vi "test-quintic-spline-04.vi"() -> ()   [LabVIEW 2019]
uses:
  <vilib>/Rock Robotics/WPI/ThirdParty/JAS_Junk/TrajLib/POSEwCURVATURE.ctl
  <vilib>/Rock Robotics/WPI/ThirdParty/JAS_Junk/TrajLib/POSE2D.ctl
  <vilib>/Rock Robotics/WPI/ThirdParty/JAS_Junk/TrajLib/TRANSLATION2D.ctl
  <vilib>/Rock Robotics/WPI/ThirdParty/JAS_Junk/TrajLib/ROTATION2D.ctl
  <vilib>/Rock Robotics/WPI/ThirdParty/JAS_Junk/TrajLib/Rotation_CreateAngle.vi
  <vilib>/Rock Robotics/WPI/ThirdParty/JAS_Junk/TrajLib/Translation_Create.vi
  <vilib>/Rock Robotics/WPI/ThirdParty/JAS_Junk/TrajLib/Util_CalcDist.vi
  <vilib>/Rock Robotics/WPI/ThirdParty/JAS_Junk/TrajLib/Trajectory_Library.lvlib
panel:
  out "XY Graph":cluster{dbl[], dbl[]}(graph)
  out "Numb\nWaypoints":i32
  out "All Interior \nwayPoints\nFound (True)":bool
  out "end rot = 0":dbl
  out "end y = 0":dbl
  out "end x = 0":dbl
  out "start rot = 0":dbl
  out "start y = 0":dbl
  out "start x = 0":dbl
  out "max dtheta < 0.0872":dbl
  out "max dy < 0.00127":dbl
  out "max dx  < 0.127":dbl
  out "Overall Error":errorcluster
  out "Elements":i32
  out "Create Spline Error":errorcluster
  out "SplinePoses\nWCurve":T1[](array[typedef]) {"POSE"."ROTATION"."SIN" format="%13.4f"; "POSE"."ROTATION"."COS" format="%13.4f"; "POSE"."ROTATION"."VALUE" format="%13.4f"; "POSE"."TRANSLATION"."Y" format="%14.3f"; "POSE"."TRANSLATION"."X" format="%14.3f"}
  out "Elapsed Time":dbl
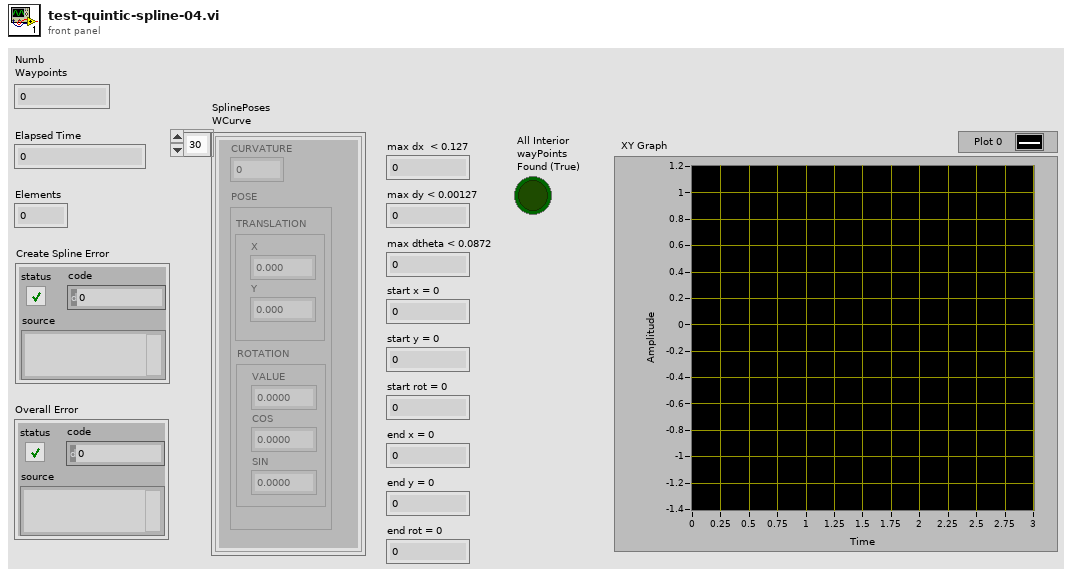
[diagram p1: front panel]
types:
  T1 = typedef "Trajectory_Library.lvlib/POSEwCURVATURE.ctl" = cluster{"CURVATURE":dbl, "POSE":T2}
  T2 = typedef "Trajectory_Library.lvlib/POSE2D.ctl" = cluster{"TRANSLATION":T3, "ROTATION":T4}
  T3 = typedef "Trajectory_Library.lvlib/TRANSLATION2D.ctl" = cluster{"X":dbl, "Y":dbl}
  T4 = typedef "Trajectory_Library.lvlib/ROTATION2D.ctl" = cluster{"VALUE":dbl, "COS":dbl, "SIN":dbl}
  T5 = typedef "Trajectory_Library.lvlib/SPLINE_CTRL_VECTOR.ctl" = cluster{"Xs":dbl[], "Ys":dbl[]}
  T6 = typedef "Trajectory_Library.lvlib/SPLINE.ctl" = cluster{"Degree":i32, "Coefficients":T7}
  T7 = typedef "NI_Matrix.lvlib/RealMatrix.ctl" = dbl[][]
  T8 = typedef "Trajectory_Library.lvlib/TWIST2D.ctl" = cluster{"dX":dbl, "dY":dbl, "dTHETA":dbl}
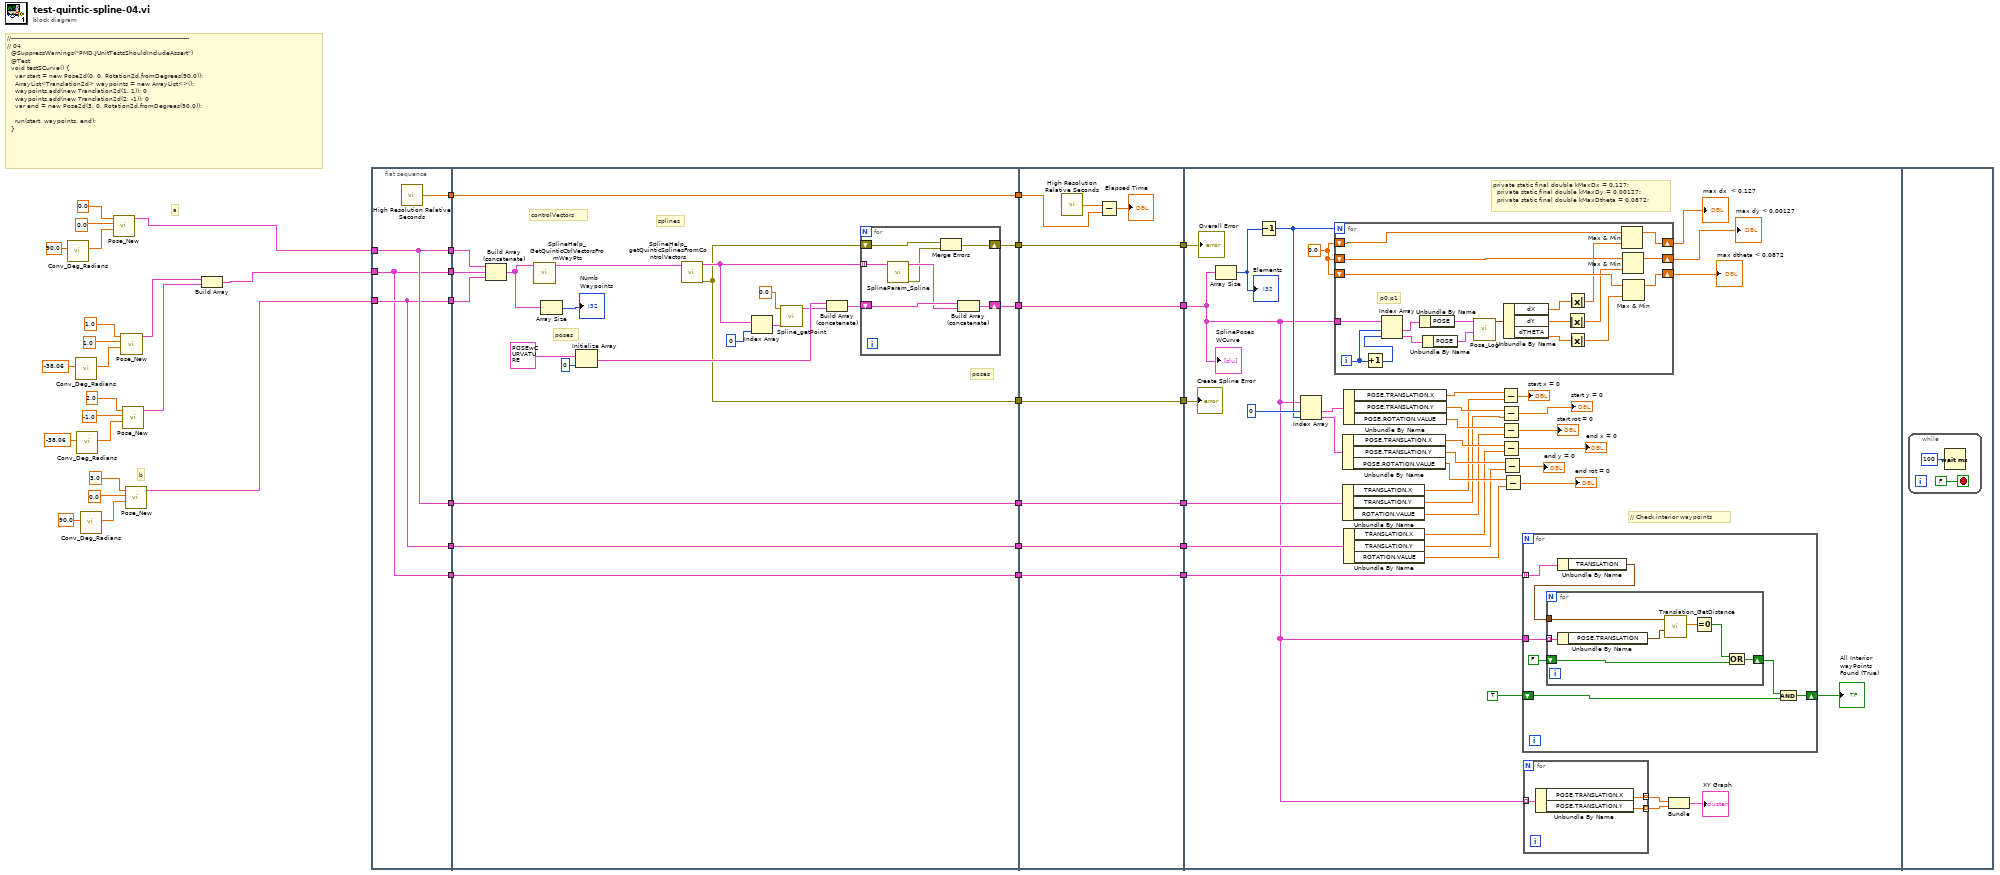
[diagram p0: block diagram]
diagram:
  # "b"
  # "a"
  # "//-----------------------------------------------------------------------------------------\n// 04\n  @SuppressWarnings(\"PMD.JUnitTestsShouldIncludeAssert\")\n  @Test\n  void testSCurve() {\n    var start = new Pose2d(0, 0, Rotation2d.fromDegrees(90.0));\n    ArrayList<Translation2d> waypoints = new ArrayList<>();\n    waypoints.add(new Translation2d(1, 1)); 0\n    waypoints.add(new Translation2d(2, -1)); 0\n    var end = new Pose2d(3, 0, Rotation2d.fromDegrees(90.0));\n\n    run(start, waypoints, end);\n  }"
  n1 = call <vilib>:"Conv_Deg_Radians.vi"("Degress"=90.0) -> ("Radians"=w15:dbl)  [unwired: 10 in]
  n2 = call <vilib>:"Conv_Deg_Radians.vi"("Degress"=-38.06) -> ("Radians"=w8:dbl)  [unwired: 10 in]
  n3 = call <vilib>:"Conv_Deg_Radians.vi"("Degress"=-38.06) -> ("Radians"=w4:dbl)  [unwired: 10 in]
  n4 = call <vilib>:"Conv_Deg_Radians.vi"("Degress"=90.0) -> ("Radians"=w18:dbl)  [unwired: 10 in]
  n5 = call <vilib>:"Pose_New.vi"("Heading"=w15, "Y"=0.0, "X"=0.0) -> ("out POSe"=w12:T2)  [unwired: 8 in]
  n6 = call <vilib>:"Pose_New.vi"("Heading"=w8, "Y"=1.0, "X"=1.0) -> ("out POSe"=w2:T2)  [unwired: 8 in]
  n7 = call <vilib>:"Pose_New.vi"("Heading"=w4, "Y"=-1.0, "X"=2.0) -> ("out POSe"=w1:T2)  [unwired: 8 in]
  n8 = call <vilib>:"Pose_New.vi"("Heading"=w18, "Y"=0.0, "X"=3.0) -> ("out POSe"=w40:T2)  [unwired: 8 in]
  n9 = Build Array(w2, w1) -> (w11:T2[])
  n10 = flat-sequence {
    tunnel: w12 -> [w44]
    tunnel: [w44] -> w41
    tunnel: w40 -> [w43]
    tunnel: [w43] -> w39
    tunnel: [w45] -> w38
    tunnel: [w44] -> w30
    tunnel: [w43] -> w27
    tunnel: [w42] -> w22
    tunnel: w11 -> [w42]
    tunnel: [w42] -> w21
    tunnel: w41 -> [w51]
    tunnel: w39 -> [w49]
    tunnel: [w67] -> w37
    tunnel: w38 -> [w67]
    tunnel: [w57] -> w36
    tunnel: [w56] -> w34
    tunnel: [w55] -> w32
    tunnel: w30 -> [w54]
    tunnel: [w54] -> w29
    tunnel: w27 -> [w53]
    tunnel: [w53] -> w26
    tunnel: [w52] -> w23
    tunnel: w22 -> [w52]
    tunnel: w21 -> [w48]
    tunnel: w37 -> [w83]
    tunnel: w36 -> [w82]
    tunnel: [w82] -> w35
    tunnel: w34 -> [w81]
    tunnel: [w81] -> w33
    tunnel: w32 -> [w80]
    tunnel: [w80] -> w31
    tunnel: w29 -> [w77]
    tunnel: [w77] -> w28
    tunnel: w26 -> [w76]
    tunnel: [w76] -> w25
    tunnel: [w75] -> w24
    tunnel: w23 -> [w75]
    tunnel: w35 -> [w85]
    tunnel: w33 -> [w121]
    tunnel: w31 -> [w120]
    tunnel: w28 -> [w114]
    tunnel: w25 -> [w113]
    tunnel: w24 -> [w90]
    frame #0 {
      n11 = call <vilib>:"High Resolution Relative Seconds.vi"() -> ("relative seconds"=w45:dbl)
    }
    frame #1 {
      # "poses"
      # "poses"
      # "splines"
      # "controlVectors"
      n12 = Build Array (concatenate)(w51, w48, w49) -> (w47:T2[])
      n13 = call <vilib>:"SplineHelp_GetQuinticCtrlVectorsFromWayPts.vi"("WayPoints"=w47) -> ("SplineControlVectors"=w50:T5[])  [unwired: 10 in]
      n14 = Array Size(array=w47) -> (size(s)=→"Numb\nWaypoints":i32)
      n15 = Initialize Array(T1 {"CURVATURE"=0.0, "POSE"={"TRANSLATION"={"X"=0.0, "Y"=0.0}, "ROTATION"={"VALUE"=0.0, "COS"=1.0, "SIN"=0.0}}} ("POSEwCURVATURE"), 0 ("dimension size")) -> (w61:T1[])
      n16 = call <vilib>:"SplineHelp_getQuinticSplinesFromControlVectors.vi"("ControlVectors"=w50) -> ("error out"=w56:errorcluster, "splines"=w58:T6[])  [unwired: 9 in]
      n17 = Index Array(array=w58, index=0) -> (element=w63:T6)
      n18 = call <vilib>:"Spline_getPoint.vi"("inputSPLINE"=w63, "Time"=0.0) -> ("POSEwCURVATURE"=w60:T1)  [unwired: 9 in]
      n19 = Build Array (concatenate)(w61, w60) -> (w59:T1[])
      n20 = for {
        shift-right: [w71] -> w57
        shift-left: w59 -> [w73]
        tunnel: w58 -> [w74] mode=indexing
        shift-right: [w69] -> w55
        shift-left: w56 -> [w70]
        n21 = call <vilib>:"SplineParam_Spline.vi"("inputSPLINE"=w74) -> ("error out"=w68:errorcluster, "outputPOSEwCURVATURE"=w72:T1[])  [unwired: 9 in]
        n22 = Merge Errors(w70, w68) -> (w69:errorcluster)
        n23 = Build Array (concatenate)(w73, w72) -> (w71:T1[])
      }
    }
    frame #2 {
      n24 = call <vilib>:"High Resolution Relative Seconds.vi"() -> ("relative seconds"=w78:dbl)
      n25 = Subtract(x=w78, y=w83) -> (x-y=→"Elapsed Time":dbl)
    }
    frame #3 {
      w118 = 0.0
      # "// Check interior waypoints"
      # "private static final double kMaxDx = 0.127;\n  private static final double kMaxDy = 0.00127;\n  private static final double kMaxDtheta = 0.0872;"
      n26 = Array Size(array=w85) -> (size(s)=w119:i32)
      "Elements" <- w119
      n27 = Decrement(x=w119) -> (x-1=w111:i32)
      n28 = Index Array(array=w85, index #1=0 ("index"), index #2=w111) -> (element #1=w110:T1, element #2=w109:T1)
      n29 = for {
        N: w111 -> [_]
        tunnel: w85 -> [w156]
        shift-right: [w147] -> w117
        shift-left: w118 -> [w144]
        shift-right: [w145] -> w115
        shift-left: w118 -> [w142]
        shift-right: [w146] -> w116
        shift-left: w118 -> [w143]
        i -> [w158]
        # "p0,p1"
        n30 = Increment(x=w158) -> (x+1=w157:i32)
        n31 = Index Array(array=w156, index #1=w158, index #2=w157) -> (element #1=w155:T1, element #2=w154:T1)
        n32 = Unbundle By Name(w155) -> ("POSE"=w153:T2)
        n33 = Unbundle By Name(w154) -> ("POSE"=w152:T2)
        n34 = call <vilib>:"Pose_Log.vi"("end POSE"=w152, "in POSE"=w153) -> ("out TWIST"=w151:T8)  [unwired: 9 in]
        n35 = Unbundle By Name(w151) -> ("dX"=w148:dbl, "dY"=w149:dbl, "dTHETA"=w150:dbl)
        n36 = Absolute Value(x=w149) -> (abs(x)=w140:dbl)
        n37 = Absolute Value(x=w148) -> (abs(x)=w141:dbl)
        n38 = Absolute Value(x=w150) -> (abs(x)=w139:dbl)
        n39 = Max & Min(x=w144, y=w141) -> (max(x,y)=w147:dbl)  [unwired: 1 out]
        n40 = Max & Min(x=w143, y=w140) -> (max(x,y)=w146:dbl)  [unwired: 1 out]
        n41 = Max & Min(x=w142, y=w139) -> (max(x,y)=w145:dbl)  [unwired: 1 out]
      }
      "max dx  < 0.127" <- w117
      "max dy < 0.00127" <- w116
      "max dtheta < 0.0872" <- w115
      n42 = Unbundle By Name(w109) -> ("POSE.TRANSLATION.X"=w105:dbl, "POSE.TRANSLATION.Y"=w104:dbl, "POSE.ROTATION.VALUE"=w103:dbl)
      n43 = Unbundle By Name(w114) -> ("TRANSLATION.X"=w102:dbl, "TRANSLATION.Y"=w101:dbl, "ROTATION.VALUE"=w100:dbl)
      n44 = Unbundle By Name(w110) -> ("POSE.TRANSLATION.X"=w108:dbl, "POSE.TRANSLATION.Y"=w107:dbl, "POSE.ROTATION.VALUE"=w106:dbl)
      n45 = Unbundle By Name(w113) -> ("TRANSLATION.X"=w99:dbl, "TRANSLATION.Y"=w98:dbl, "ROTATION.VALUE"=w97:dbl)
      n46 = Subtract(x=w108, y=w102) -> (x-y=→"start x = 0":dbl)
      n47 = Subtract(x=w107, y=w101) -> (x-y=→"start y = 0":dbl)
      n48 = Subtract(x=w106, y=w100) -> (x-y=→"start rot = 0":dbl)
      n49 = Subtract(x=w105, y=w99) -> (x-y=→"end x = 0":dbl)
      n50 = Subtract(x=w104, y=w98) -> (x-y=→"end y = 0":dbl)
      n51 = Subtract(x=w103, y=w97) -> (x-y=→"end rot = 0":dbl)
      n52 = for {
        tunnel: w90 -> [w126] mode=indexing
        tunnel: w85 -> [w131]
        shift-right: [w130] -> w88
        shift-left: TRUE -> [w129]
        n53 = Unbundle By Name(w126) -> ("TRANSLATION"=w125:T3)
        n54 = for {
          tunnel: w131 -> [w135] mode=indexing
          shift-right: [w138] -> w127
          shift-left: FALSE -> [w137]
          tunnel: w125 -> [w136]
          n55 = Unbundle By Name(w135) -> ("POSE.TRANSLATION"=w134:T3)
          n56 = call <vilib>:"Translation_GetDistance.vi"("other Translation"=w134, "In Translation"=w136) -> ("Distance"=w133:dbl)  [unwired: 9 in]
          n57 = Equal To 0?(x=w133) -> (x = 0?=w132:bool)
          n58 = Or(x=w132, y=w137) -> (x .or. y?=w138:bool)
        }
        n59 = And(x=w127, y=w129) -> (x .and. y?=w130:bool)
      }
      "All Interior \nwayPoints\nFound (True)" <- w88
      n60 = for {
        tunnel: [w124] -> w87 mode=indexing
        tunnel: [w123] -> w86 mode=indexing
        tunnel: w85 -> [w122] mode=indexing
        n61 = Unbundle By Name(w122) -> ("POSE.TRANSLATION.X"=w124:dbl, "POSE.TRANSLATION.Y"=w123:dbl)
      }
      n62 = Bundle(w87, w86) -> (→"XY Graph":cluster{dbl[], dbl[]})  [unwired: 1 in]
      "SplinePoses\nWCurve" <- w85
      "Create Spline Error" <- w121
      "Overall Error" <- w120
    }
    frame #4 {
      n63 = while {
        stop <- FALSE stop-if-true
        n64 = Wait (ms)(milliseconds to wait=u32 100) -> ()  [unwired: 1 out]
      }
    }
  }
